vi "CRY6175SwitchAPI.vi"(9 "Parameter":string, 11 "Function Name":string) -> (3 "bResult":bool)   [LabVIEW 2013]
uses:
  CRY6175APT_Win32.dll
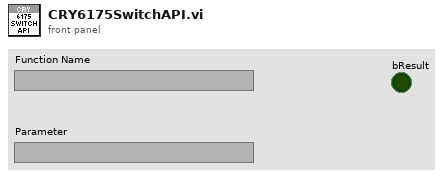
[diagram p1: front panel]
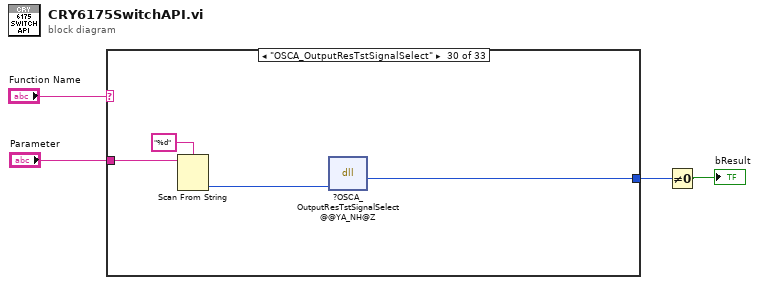
[diagram p0: block diagram]
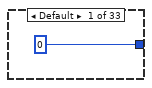
[diagram p2: hidden frame]
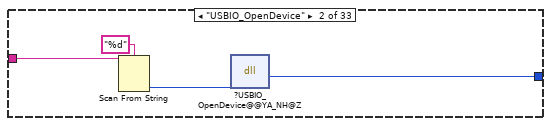
[diagram p3: hidden frame]
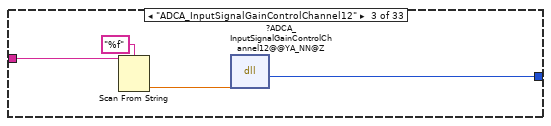
[diagram p4: hidden frame]
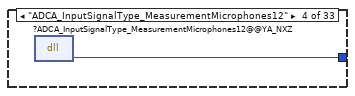
[diagram p5: hidden frame]
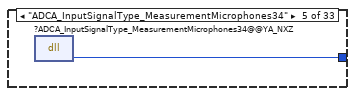
[diagram p6: hidden frame]
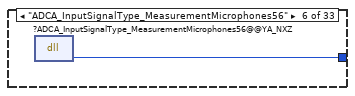
[diagram p7: hidden frame]
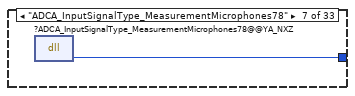
[diagram p8: hidden frame]
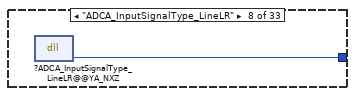
[diagram p9: hidden frame]
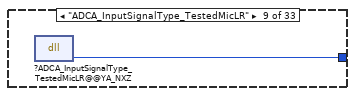
[diagram p10: hidden frame]
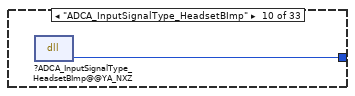
[diagram p11: hidden frame]
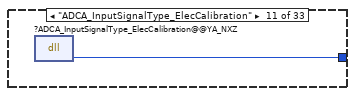
[diagram p12: hidden frame]
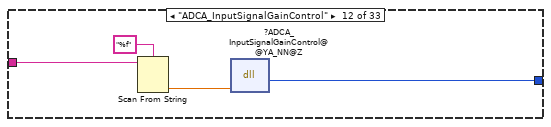
[diagram p13: hidden frame]
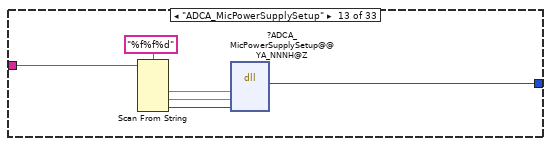
[diagram p14: hidden frame]
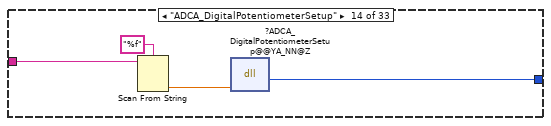
[diagram p15: hidden frame]
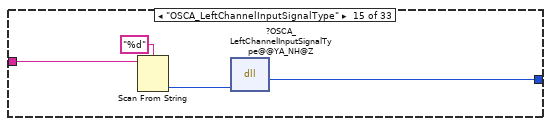
[diagram p16: hidden frame]
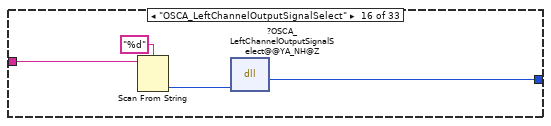
[diagram p17: hidden frame]
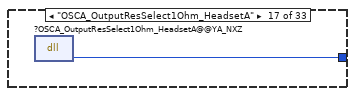
[diagram p18: hidden frame]
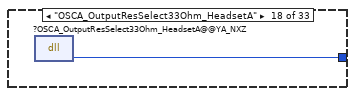
[diagram p19: hidden frame]
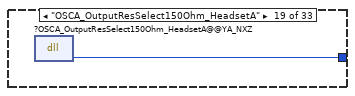
[diagram p20: hidden frame]
diagram:
  n1 = case shown="\"OSCA_OutputResTstSignalSelect\"" "Function Name" {
    tunnel: "Parameter" -> [_ w7 w11 _ _ _ _ _ _ _ _ w23 w29 w33 w37 w41 _ _ _ _ _ _ _ w52 w56 w60 w64 w68 w72 w76 w80 _ _]
    tunnel: [0 ("return type") w9 w13 w14 w15 w16 w17 w18 w19 w20 w21 w25 w31 w35 w39 w43 w44 w45 w46 w47 w48 w49 w50 w54 w58 w62 w66 w70 w74 w78 w82 w83 w84] -> w2
    frame Default {
    }
    frame "USBIO_OpenDevice" {
      n2 = Scan From String(format string="%d", input string=w7) -> (output 1=w6:i32)  [unwired: 3 in, 3 out]
      n3 = dll-call lib="D:/LabView_Project/CRY6181/CRYSystem/Hardware/SubVI/CRY6175APT_Win32.dll" fn="?USBIO_OpenDevice@@YA_NH@Z"("nDevID"=w6) -> ("return type"=w9:i32)  [unwired: 4 in, 2 out]
    }
    frame "ADCA_InputSignalGainControlChannel12" {
      n4 = Scan From String(format string="%f", input string=w11) -> (output 1=w10:dbl)  [unwired: 3 in, 3 out]
      n5 = dll-call lib="D:/LabView_Project/CRY6181/CRYSystem/Hardware/SubVI/CRY6175APT_Win32.dll" fn="?ADCA_InputSignalGainControlChannel12@@YA_NN@Z"("dTotalGain"=w10) -> ("return type"=w13:i32)  [unwired: 4 in, 2 out]
    }
    frame "ADCA_InputSignalType_MeasurementMicrophones12" {
      n6 = dll-call lib="D:/LabView_Project/CRY6181/CRYSystem/Hardware/SubVI/CRY6175APT_Win32.dll" fn="?ADCA_InputSignalType_MeasurementMicrophones12@@YA_NXZ"() -> ("return type"=w14:i32)  [unwired: 3 in, 2 out]
    }
    frame "ADCA_InputSignalType_MeasurementMicrophones34" {
      n7 = dll-call lib="D:/LabView_Project/CRY6181/CRYSystem/Hardware/SubVI/CRY6175APT_Win32.dll" fn="?ADCA_InputSignalType_MeasurementMicrophones34@@YA_NXZ"() -> ("return type"=w15:i32)  [unwired: 3 in, 2 out]
    }
    frame "ADCA_InputSignalType_MeasurementMicrophones56" {
      n8 = dll-call lib="D:/LabView_Project/CRY6181/CRYSystem/Hardware/SubVI/CRY6175APT_Win32.dll" fn="?ADCA_InputSignalType_MeasurementMicrophones56@@YA_NXZ"() -> ("return type"=w16:i32)  [unwired: 3 in, 2 out]
    }
    frame "ADCA_InputSignalType_MeasurementMicrophones78" {
      n9 = dll-call lib="D:/LabView_Project/CRY6181/CRYSystem/Hardware/SubVI/CRY6175APT_Win32.dll" fn="?ADCA_InputSignalType_MeasurementMicrophones78@@YA_NXZ"() -> ("return type"=w17:i32)  [unwired: 3 in, 2 out]
    }
    frame "ADCA_InputSignalType_LineLR" {
      n10 = dll-call lib="D:/LabView_Project/CRY6181/CRYSystem/Hardware/SubVI/CRY6175APT_Win32.dll" fn="?ADCA_InputSignalType_LineLR@@YA_NXZ"() -> ("return type"=w18:i32)  [unwired: 3 in, 2 out]
    }
    frame "ADCA_InputSignalType_TestedMicLR" {
      n11 = dll-call lib="D:/LabView_Project/CRY6181/CRYSystem/Hardware/SubVI/CRY6175APT_Win32.dll" fn="?ADCA_InputSignalType_TestedMicLR@@YA_NXZ"() -> ("return type"=w19:i32)  [unwired: 3 in, 2 out]
    }
    frame "ADCA_InputSignalType_HeadsetBImp" {
      n12 = dll-call lib="D:/LabView_Project/CRY6181/CRYSystem/Hardware/SubVI/CRY6175APT_Win32.dll" fn="?ADCA_InputSignalType_HeadsetBImp@@YA_NXZ"() -> ("return type"=w20:i32)  [unwired: 3 in, 2 out]
    }
    frame "ADCA_InputSignalType_ElecCalibration" {
      n13 = dll-call lib="D:/LabView_Project/CRY6181/CRYSystem/Hardware/SubVI/CRY6175APT_Win32.dll" fn="?ADCA_InputSignalType_ElecCalibration@@YA_NXZ"() -> ("return type"=w21:i32)  [unwired: 3 in, 2 out]
    }
    frame "ADCA_InputSignalGainControl" {
      n14 = Scan From String(format string="%f", input string=w23) -> (output 1=w22:dbl)  [unwired: 3 in, 3 out]
      n15 = dll-call lib="D:/LabView_Project/CRY6181/CRYSystem/Hardware/SubVI/CRY6175APT_Win32.dll" fn="?ADCA_InputSignalGainControl@@YA_NN@Z"("dTotalGain"=w22) -> ("return type"=w25:i32)  [unwired: 4 in, 2 out]
    }
    frame "ADCA_MicPowerSupplySetup" {
      n16 = Scan From String(format string="%f%f%d", input string=w29) -> (output 1=w28:dbl, output 2=w27:dbl, output 3=w26:i32)  [unwired: 5 in, 3 out]
      n17 = dll-call lib="D:/LabView_Project/CRY6181/CRYSystem/Hardware/SubVI/CRY6175APT_Win32.dll" fn="?ADCA_MicPowerSupplySetup@@YA_NNNH@Z"("dMicVoltageL"=w28, "dMicVoltageR"=w27, "eChannelsType"=w26) -> ("return type"=w31:i32)  [unwired: 6 in, 2 out]
    }
    frame "ADCA_DigitalPotentiometerSetup" {
      n18 = Scan From String(format string="%f", input string=w33) -> (output 1=w32:dbl)  [unwired: 3 in, 3 out]
      n19 = dll-call lib="D:/LabView_Project/CRY6181/CRYSystem/Hardware/SubVI/CRY6175APT_Win32.dll" fn="?ADCA_DigitalPotentiometerSetup@@YA_NN@Z"("dRes"=w32) -> ("return type"=w35:i32)  [unwired: 4 in, 2 out]
    }
    frame "OSCA_LeftChannelInputSignalType" {
      n20 = Scan From String(format string="%d", input string=w37) -> (output 1=w36:i32)  [unwired: 3 in, 3 out]
      n21 = dll-call lib="D:/LabView_Project/CRY6181/CRYSystem/Hardware/SubVI/CRY6175APT_Win32.dll" fn="?OSCA_LeftChannelInputSignalType@@YA_NH@Z"("eSignalType"=w36) -> ("return type"=w39:i32)  [unwired: 4 in, 2 out]
    }
    frame "OSCA_LeftChannelOutputSignalSelect" {
      n22 = Scan From String(format string="%d", input string=w41) -> (output 1=w40:i32)  [unwired: 3 in, 3 out]
      n23 = dll-call lib="D:/LabView_Project/CRY6181/CRYSystem/Hardware/SubVI/CRY6175APT_Win32.dll" fn="?OSCA_LeftChannelOutputSignalSelect@@YA_NH@Z"("eOutputSignalType"=w40) -> ("return type"=w43:i32)  [unwired: 4 in, 2 out]
    }
    frame "OSCA_OutputResSelect1Ohm_HeadsetA" {
      n24 = dll-call lib="D:/LabView_Project/CRY6181/CRYSystem/Hardware/SubVI/CRY6175APT_Win32.dll" fn="?OSCA_OutputResSelect1Ohm_HeadsetA@@YA_NXZ"() -> ("return type"=w44:i32)  [unwired: 3 in, 2 out]
    }
    frame "OSCA_OutputResSelect33Ohm_HeadsetA" {
      n25 = dll-call lib="D:/LabView_Project/CRY6181/CRYSystem/Hardware/SubVI/CRY6175APT_Win32.dll" fn="?OSCA_OutputResSelect33Ohm_HeadsetA@@YA_NXZ"() -> ("return type"=w45:i32)  [unwired: 3 in, 2 out]
    }
    frame "OSCA_OutputResSelect150Ohm_HeadsetA" {
      n26 = dll-call lib="D:/LabView_Project/CRY6181/CRYSystem/Hardware/SubVI/CRY6175APT_Win32.dll" fn="?OSCA_OutputResSelect150Ohm_HeadsetA@@YA_NXZ"() -> ("return type"=w46:i32)  [unwired: 3 in, 2 out]
    }
    frame "OSCA_OutputResSelect600Ohm_HeadsetA" {
      n27 = dll-call lib="D:/LabView_Project/CRY6181/CRYSystem/Hardware/SubVI/CRY6175APT_Win32.dll" fn="?OSCA_OutputResSelect600Ohm_HeadsetA@@YA_NXZ"() -> ("return type"=w47:i32)  [unwired: 3 in, 2 out]
    }
    frame "OSCA_OutputResSelect750Ohm_HeadsetA" {
      n28 = dll-call lib="D:/LabView_Project/CRY6181/CRYSystem/Hardware/SubVI/CRY6175APT_Win32.dll" fn="?OSCA_OutputResSelect750Ohm_HeadsetA@@YA_NXZ"() -> ("return type"=w48:i32)  [unwired: 3 in, 2 out]
    }
    frame "OSCA_OutputResSelect1Ohm_HeadsetB" {
      n29 = dll-call lib="D:/LabView_Project/CRY6181/CRYSystem/Hardware/SubVI/CRY6175APT_Win32.dll" fn="?OSCA_OutputResSelect1Ohm_HeadsetB@@YA_NXZ"() -> ("return type"=w49:i32)  [unwired: 3 in, 2 out]
    }
    frame "OSCA_OutputResSelect33Ohm_HeadsetB" {
      n30 = dll-call lib="D:/LabView_Project/CRY6181/CRYSystem/Hardware/SubVI/CRY6175APT_Win32.dll" fn="?OSCA_OutputResSelect33Ohm_HeadsetB@@YA_NXZ"() -> ("return type"=w50:i32)  [unwired: 3 in, 2 out]
    }
    frame "OSCA_ArtificialMouthOutput" {
      n31 = Scan From String(format string="%d", input string=w52) -> (output 1=w51:i32)  [unwired: 3 in, 3 out]
      n32 = dll-call lib="D:/LabView_Project/CRY6181/CRYSystem/Hardware/SubVI/CRY6175APT_Win32.dll" fn="?OSCA_ArtificialMouthOutput@@YA_NH@Z"("eArtificialMouthIndex"=w51) -> ("return type"=w54:i32)  [unwired: 4 in, 2 out]
    }
    frame "ADCA_InputSignalSelect_N239" {
      n33 = Scan From String(format string="%d", input string=w56) -> (output 1=w55:i32)  [unwired: 3 in, 3 out]
      n34 = dll-call lib="D:/LabView_Project/CRY6181/CRYSystem/Hardware/SubVI/CRY6175APT_Win32.dll" fn="?ADCA_InputSignalSelect_N239@@YA_NH@Z"("eSignalSel"=w55) -> ("return type"=w58:i32)  [unwired: 4 in, 2 out]
    }
    frame "ADCA_InputSignalSelect_N231" {
      n35 = Scan From String(format string="%d", input string=w60) -> (output 1=w59:i32)  [unwired: 3 in, 3 out]
      n36 = dll-call lib="D:/LabView_Project/CRY6181/CRYSystem/Hardware/SubVI/CRY6175APT_Win32.dll" fn="?ADCA_InputSignalSelect_N231@@YA_NH@Z"("eSignalSel"=w59) -> ("return type"=w62:i32)  [unwired: 4 in, 2 out]
    }
    frame "ADCA_InputSignalSelect_N246" {
      n37 = Scan From String(format string="%d", input string=w64) -> (output 1=w63:i32)  [unwired: 3 in, 3 out]
      n38 = dll-call lib="D:/LabView_Project/CRY6181/CRYSystem/Hardware/SubVI/CRY6175APT_Win32.dll" fn="?ADCA_InputSignalSelect_N246@@YA_NH@Z"("eSignalSel"=w63) -> ("return type"=w66:i32)  [unwired: 4 in, 2 out]
    }
    frame "ADCA_StopModulationSignal" {
      n39 = Scan From String(format string="%d", input string=w68) -> (output 1=w67:i32)  [unwired: 3 in, 3 out]
      n40 = dll-call lib="D:/LabView_Project/CRY6181/CRYSystem/Hardware/SubVI/CRY6175APT_Win32.dll" fn="?ADCA_StopModulationSignal@@YA_NH@Z"("eChipSel"=w67) -> ("return type"=w70:i32)  [unwired: 4 in, 2 out]
    }
    frame "ADCA_StartModulationSignal" {
      n41 = Scan From String(format string="%d", input string=w72) -> (output 1=w71:i32)  [unwired: 3 in, 3 out]
      n42 = dll-call lib="D:/LabView_Project/CRY6181/CRYSystem/Hardware/SubVI/CRY6175APT_Win32.dll" fn="?ADCA_StartModulationSignal@@YA_NH@Z"("eChipSel"=w71) -> ("return type"=w74:i32)  [unwired: 4 in, 2 out]
    }
    frame "OSCA_OutputResTstSignalSelect" {
      n43 = Scan From String(format string="%d", input string=w76) -> (output 1=w75:i32)  [unwired: 3 in, 3 out]
      n44 = dll-call lib="D:/LabView_Project/CRY6181/CRYSystem/Hardware/SubVI/CRY6175APT_Win32.dll" fn="?OSCA_OutputResTstSignalSelect@@YA_NH@Z"("eOutputSignalSel"=w75) -> ("return type"=w78:i32)  [unwired: 4 in, 2 out]
    }
    frame "ADCA_InputSignalGainControl_N235" {
      n45 = Scan From String(format string="%f", input string=w80) -> (output 1=w79:dbl)  [unwired: 3 in, 3 out]
      n46 = dll-call lib="D:/LabView_Project/CRY6181/CRYSystem/Hardware/SubVI/CRY6175APT_Win32.dll" fn="?ADCA_InputSignalGainControl_N235@@YA_NN@Z"("dRatio"=w79) -> ("return type"=w82:i32)  [unwired: 4 in, 2 out]
    }
    frame "GetCompanyLogo" {
      n47 = dll-call lib="D:/LabView_Project/CRY6181/CRYSystem/Hardware/SubVI/CRY6175APT_Win32.dll" fn="?GetCompanyLogo@@YA_NXZ"() -> ("return type"=w83:i32)  [unwired: 3 in, 2 out]
    }
    frame "CheckOutSequence" {
      n48 = dll-call lib="D:/LabView_Project/CRY6181/CRYSystem/Hardware/SubVI/CRY6175APT_Win32.dll" fn="?CheckOutSequence@@YA_NXZ"() -> ("return type"=w84:i32)  [unwired: 3 in, 2 out]
    }
  }
  n49 = Not Equal To 0?(x=w2) -> (x != 0?=→"bResult":bool)
